vi "Open Talon Brtrfly v2.vi"() -> ()   [LabVIEW 2018]
uses:
  <vilib>/Rock Robotics/WPI/ThirdParty/Phoenix-LabVIEW/Motor Controller/Controls/CTRE_Phoenix_MotorControl_NeutralMode.ctl
  <vilib>/Rock Robotics/WPI/ThirdParty/Phoenix-LabVIEW/Motor Controller/Controls/CTRE_Phoenix_MotorControl_ControlMode.ctl
panel:
  out "Cursor.Cursor Position:Cursor Y":dbl
  out "Cursor.Cursor Position:Cursor X":dbl
  in  "Digital Joystick":cluster{"X":dbl, "Y":dbl}[](graph)
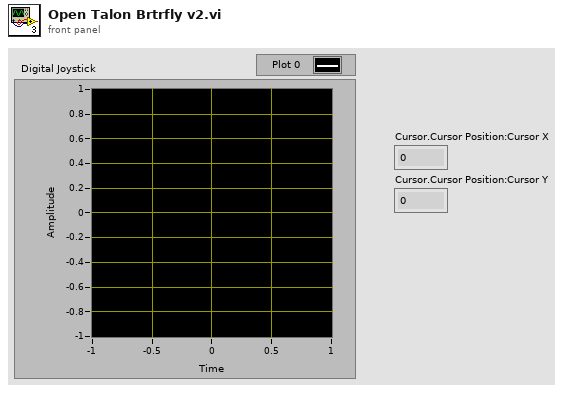
[diagram p1: front panel]
types:
  T1 = typedef "CTRE_Phoenix_MotorControl_ControlMode.ctl" = u16
  T2 = typedef "CTRE_Phoenix_MotorControl_NeutralMode.ctl" = enum8{"EEPROMSetting", "Override to Coast", "Override to Brake"}
  T3 = enum16{"FollowerType_PercentOutput", "FollowerType_AuxOutput1"}
  T4 = typedef "WPI_MotorControlDeviceRef.ctl" = cluster{"DeviceStatus":errorcluster, "Type":T5, "PWM":cluster{"PWM Channel":T6, "DeadBand":T7}, "CAN":cluster{"Device Number":u8, "SetOutput VI Ref":variant, "GetOutput VI Ref":variant, "Enable VI Ref":variant, "Disable VI Ref":variant, "Data":variant}, "Invert":bool, "DIO PWM":cluster{"PWM \"Enable\" Channel":T6, "DIOChannel":T8, "PWM Rate":dbl}}
  T5 = typedef "WPI_MotorControlType.ctl" = enum16{"PWM", "CAN", "DIO PWM"}
  T6 = typedef "FPGA_DIOPWMChannel.ctl" = enum8{"PWM 0", "PWM 1", "PWM 2", "PWM 3", "PWM 4", "PWM 5", "PWM 6", "PWM 7", "PWM 8", "PWM 9", "PWM MXP 0", "PWM MXP 1", "PWM MXP 2", "PWM MXP 3", "PWM MXP 4", "PWM MXP 5", "PWM MXP 6", "PWM MXP 7", "PWM MXP 8", "PWM MXP 9", "Invalid"}
  T7 = typedef "WPI_PWMDeadband.ctl" = cluster{"Name":string, "maxPositivePwm":i32, "minPositivePwm":i32, "centerPwm":i32, "maxNegativePwm":i32, "minNegativePwm":i32, "angularRange":u16}
  T8 = typedef "FPGA_DIOChannel.ctl" = enum8{"DIO 0", "DIO 1", "DIO 2", "DIO 3", "DIO 4", "DIO 5", "DIO 6", "DIO 7", "DIO 8", "DIO 9", "DIO MXP 0", "DIO MXP 1", "DIO MXP 2", "DIO MXP 3", "DIO MXP 4", "DIO MXP 5", "DIO MXP 6", "DIO MXP 7", "DIO MXP 8", "DIO MXP 9", "DIO MXP 10", "DIO MXP 11", "DIO MXP 12", "DIO MXP 13", "DIO MXP 14", "DIO MXP 15", "SPI Port CS1", "SPI Port CS2", "SPI Port CS3", "SPI Port MISO", "SPI Port MOSI", "Invalid"}
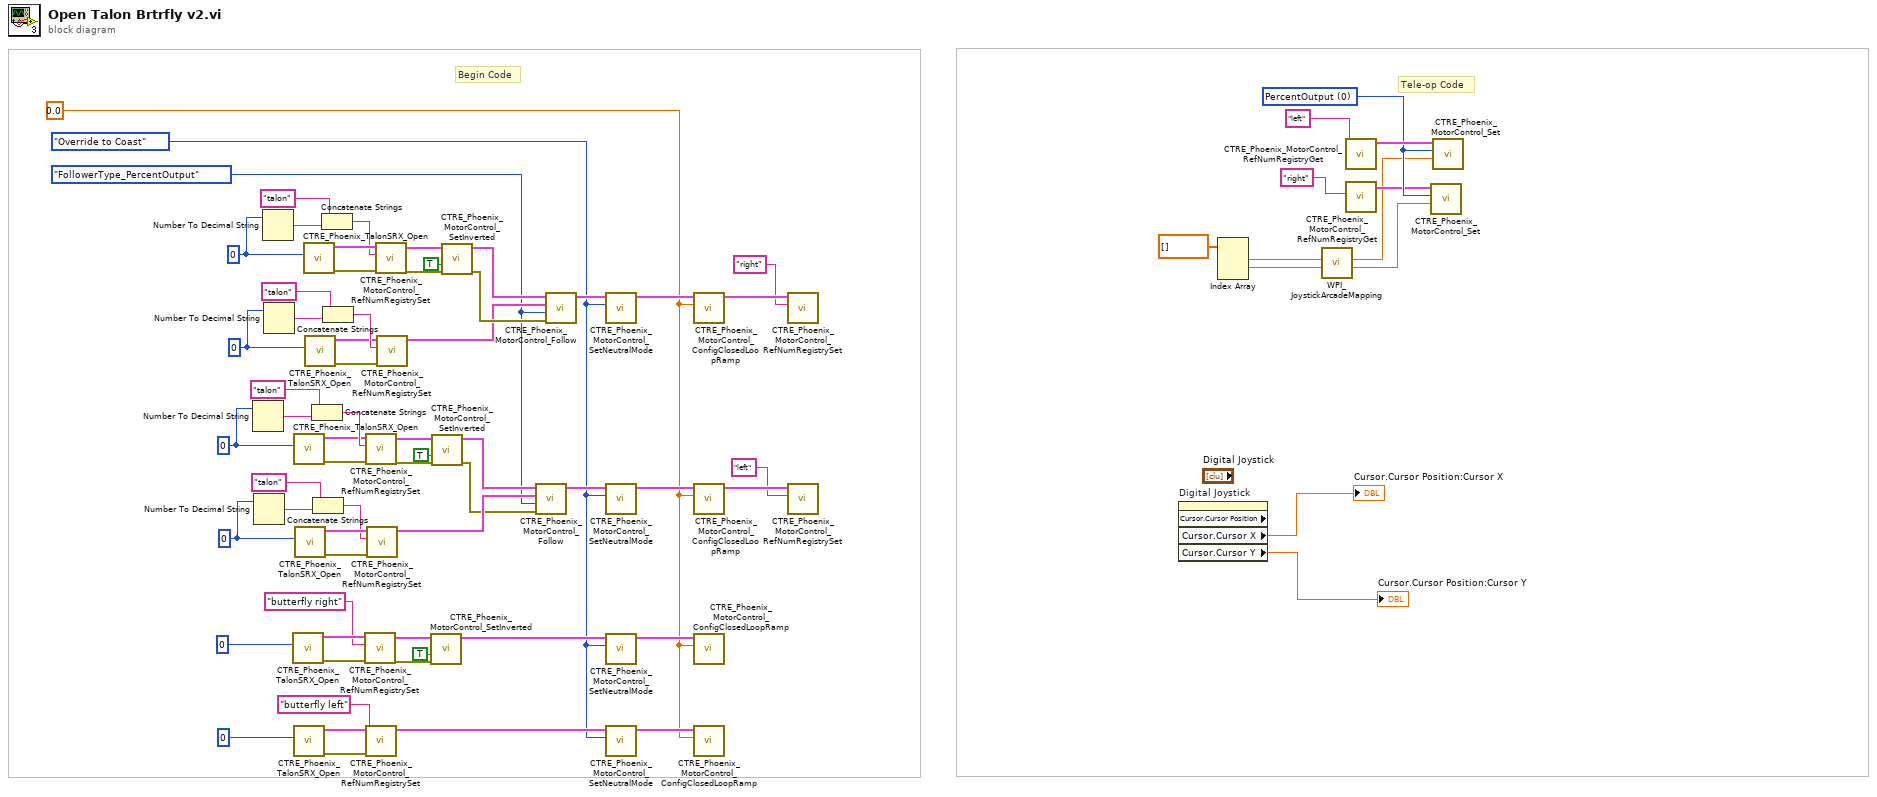
[diagram p0: block diagram]
diagram:
  w14 = T1 0 items=["PercentOutput"=0, "Position"=1, "Velocity"=2, "Current"=3, "Follower"=5, "MotionProfile"=6, "MotionMagic"=7, "MotionProfileArc"=10, "Disabled"=15] ("Control Mode")
  w2 = 0.0 ("secondsFromNeutralToFull")
  w1 = CTRE_Phoenix_MotorControl_NeutralMode."Override to Coast" ("Motor Control Neutral Mode")
  w25 = T3."FollowerType_PercentOutput" ("FollowerType")
  w47 = u8 0 ("Device Number")
  w40 = u8 0 ("Device Number")
  w62 = u8 0 ("Device Number")
  w69 = u8 0 ("Device Number")
  # "Tele-op Code"
  # "Begin Code"
  n1 = Number To Decimal String(number=w40) -> (decimal integer string=w41:string)  [unwired: 1 in]
  n2 = Number To Decimal String(number=w47) -> (decimal integer string=w46:string)  [unwired: 1 in]
  n3 = Number To Decimal String(number=w69) -> (decimal integer string=w68:string)  [unwired: 1 in]
  n4 = Number To Decimal String(number=w62) -> (decimal integer string=w63:string)  [unwired: 1 in]
  n5 = call <vilib>:"CTRE_Phoenix_TalonSRX_Open.vi"("Device Number"=u8 0) -> ("error out"=w33:errorcluster, "CAN Talon SRX Ref"=w32:T4)  [unwired: 9 in]
  n6 = call <vilib>:"CTRE_Phoenix_TalonSRX_Open.vi"("Device Number"=w40) -> ("error out"=w38:errorcluster, "CAN Talon SRX Ref"=w39:T4)  [unwired: 9 in]
  n7 = call <vilib>:"CTRE_Phoenix_TalonSRX_Open.vi"("Device Number"=u8 0) -> ("error out"=w28:errorcluster, "CAN Talon SRX Ref"=w29:T4)  [unwired: 9 in]
  n8 = call <vilib>:"CTRE_Phoenix_TalonSRX_Open.vi"("Device Number"=w47) -> ("error out"=w49:errorcluster, "CAN Talon SRX Ref"=w48:T4)  [unwired: 9 in]
  n9 = call <vilib>:"CTRE_Phoenix_TalonSRX_Open.vi"("Device Number"=w69) -> ("error out"=w71:errorcluster, "CAN Talon SRX Ref"=w70:T4)  [unwired: 9 in]
  n10 = call <vilib>:"CTRE_Phoenix_TalonSRX_Open.vi"("Device Number"=w62) -> ("error out"=w60:errorcluster, "CAN Talon SRX Ref"=w61:T4)  [unwired: 9 in]
  n11 = Concatenate Strings("talon" ("string"), w41) -> (w43:string)
  n12 = Concatenate Strings("talon" ("string"), w46) -> (w44:string)
  n13 = Concatenate Strings("talon" ("string"), w68) -> (w66:string)
  n14 = Concatenate Strings("talon" ("string"), w63) -> (w65:string)
  n15 = call <vilib>:"CTRE_Phoenix_MotorControl_RefNumRegistrySet.vi"("error in (no error)"=w33, "refnum name"="butterfly right", "PhoenixMotorControlDevRef"=w32) -> ("error out"=w26:errorcluster, "PhoenixMotorControlDevRef"=w27:T4)  [unwired: 7 in]
  n16 = call <vilib>:"CTRE_Phoenix_MotorControl_RefNumRegistrySet.vi"("error in (no error)"=w38, "refnum name"=w43, "PhoenixMotorControlDevRef"=w39) -> ("error out"=w51:errorcluster, "PhoenixMotorControlDevRef"=w50:T4)  [unwired: 7 in]
  n17 = call <vilib>:"CTRE_Phoenix_MotorControl_RefNumRegistrySet.vi"("error in (no error)"=w28, "refnum name"="butterfly left", "PhoenixMotorControlDevRef"=w29) -> ("PhoenixMotorControlDevRef"=w5:T4)  [unwired: 7 in, 1 out]
  n18 = call <vilib>:"CTRE_Phoenix_MotorControl_RefNumRegistrySet.vi"("error in (no error)"=w49, "refnum name"=w44, "PhoenixMotorControlDevRef"=w48) -> ("PhoenixMotorControlDevRef"=w54:T4)  [unwired: 7 in, 1 out]
  n19 = call <vilib>:"CTRE_Phoenix_MotorControl_RefNumRegistrySet.vi"("error in (no error)"=w71, "refnum name"=w66, "PhoenixMotorControlDevRef"=w70) -> ("error out"=w58:errorcluster, "PhoenixMotorControlDevRef"=w59:T4)  [unwired: 7 in]
  n20 = call <vilib>:"CTRE_Phoenix_MotorControl_RefNumRegistrySet.vi"("error in (no error)"=w60, "refnum name"=w65, "PhoenixMotorControlDevRef"=w61) -> ("PhoenixMotorControlDevRef"=w55:T4)  [unwired: 7 in, 1 out]
  n21 = call <vilib>:"CTRE_Phoenix_MotorControl_SetInverted.vi"("error in (no error)"=w26, "Invert?"=TRUE, "PhoenixMotorControlDevRef"=w27) -> ("PhoenixMotorControlDevRef"=w6:T4)  [unwired: 7 in, 1 out]
  n22 = call <vilib>:"CTRE_Phoenix_MotorControl_SetInverted.vi"("error in (no error)"=w51, "Invert?"=TRUE, "PhoenixMotorControlDevRef"=w50) -> ("error out"=w52:errorcluster, "PhoenixMotorControlDevRef"=w53:T4)  [unwired: 7 in]
  n23 = call <vilib>:"CTRE_Phoenix_MotorControl_SetInverted.vi"("error in (no error)"=w58, "Invert?"=TRUE, "PhoenixMotorControlDevRef"=w59) -> ("error out"=w57:errorcluster, "PhoenixMotorControlDevRef"=w56:T4)  [unwired: 7 in]
  n24 = call <vilib>:"CTRE_Phoenix_MotorControl_Follow.vi"("error in (no error)"=w52, "FollowerType"=w25, "Master Controller to Follow"=w54, "PhoenixMotorControlDevRef"=w53) -> ("PhoenixMotorControlDevRef"=w36:T4)  [unwired: 6 in, 1 out]
  n25 = call <vilib>:"CTRE_Phoenix_MotorControl_Follow.vi"("error in (no error)"=w57, "FollowerType"=w25, "Master Controller to Follow"=w55, "PhoenixMotorControlDevRef"=w56) -> ("PhoenixMotorControlDevRef"=w73:T4)  [unwired: 6 in, 1 out]
  n26 = call <vilib>:"CTRE_Phoenix_MotorControl_SetNeutralMode.vi"("Motor Control Neutral Mode"=w1, "PhoenixMotorControlDevRef"=w73) -> ("PhoenixMotorControlDevRef"=w72:T4)  [unwired: 8 in, 1 out]
  n27 = call <vilib>:"CTRE_Phoenix_MotorControl_SetNeutralMode.vi"("Motor Control Neutral Mode"=w1, "PhoenixMotorControlDevRef"=w36) -> ("PhoenixMotorControlDevRef"=w37:T4)  [unwired: 8 in, 1 out]
  n28 = call <vilib>:"CTRE_Phoenix_MotorControl_SetNeutralMode.vi"("Motor Control Neutral Mode"=w1, "PhoenixMotorControlDevRef"=w6) -> ("PhoenixMotorControlDevRef"=w3:T4)  [unwired: 8 in, 1 out]
  n29 = call <vilib>:"CTRE_Phoenix_MotorControl_SetNeutralMode.vi"("Motor Control Neutral Mode"=w1, "PhoenixMotorControlDevRef"=w5) -> ("PhoenixMotorControlDevRef"=w4:T4)  [unwired: 8 in, 1 out]
  n30 = call <vilib>:"CTRE_Phoenix_MotorControl_ConfigClosedLoopRamp.vi"("secondsFromNeutralToFull"=w2, "PhoenixMotorControlDevRef"=w72) -> ("PhoenixMotorControlDevRef"=w24:T4)  [unwired: 8 in, 1 out]
  n31 = call <vilib>:"CTRE_Phoenix_MotorControl_ConfigClosedLoopRamp.vi"("secondsFromNeutralToFull"=w2, "PhoenixMotorControlDevRef"=w37) -> ("PhoenixMotorControlDevRef"=w23:T4)  [unwired: 8 in, 1 out]
  n32 = call <vilib>:"CTRE_Phoenix_MotorControl_ConfigClosedLoopRamp.vi"("secondsFromNeutralToFull"=w2, "PhoenixMotorControlDevRef"=w3) -> ()  [unwired: 8 in, 2 out]
  n33 = call <vilib>:"CTRE_Phoenix_MotorControl_ConfigClosedLoopRamp.vi"("secondsFromNeutralToFull"=w2, "PhoenixMotorControlDevRef"=w4) -> ()  [unwired: 8 in, 2 out]
  n34 = call <vilib>:"CTRE_Phoenix_MotorControl_RefNumRegistrySet.vi"("refnum name"="right", "PhoenixMotorControlDevRef"=w24) -> ()  [unwired: 8 in, 2 out]
  n35 = call <vilib>:"CTRE_Phoenix_MotorControl_RefNumRegistrySet.vi"("refnum name"="left", "PhoenixMotorControlDevRef"=w23) -> ()  [unwired: 8 in, 2 out]
  n36 = property on="Digital Joystick" class="XYGraph (strict)" props=["Cursor", "Cursor Position", "Cursor", "Cursor X", "Cursor", "Cursor Y"]() -> ("Cursor.Cursor X"=→"Cursor.Cursor Position:Cursor X":dbl, "Cursor.Cursor Y"=→"Cursor.Cursor Position:Cursor Y":dbl)  [unwired: 2 in, 3 out]
  n37 = Index Array(array=dbl[] []) -> (element #1=w19:dbl, element #2=w18:dbl)  [unwired: 3 in, 1 out]
  n38 = call <vilib>:"WPI_JoystickArcadeMapping.vi"("Y axis value"=w18, "X axis value"=w19) -> ("Right Motor Value"=w11:dbl, "Left Motor Value"=w12:dbl)  [unwired: 8 in]
  n39 = call <vilib>:"CTRE_Phoenix_MotorControl_RefNumRegistryGet.vi"("refnum name"="left") -> ("PhoenixMotorControlDevRef"=w15:T4)  [unwired: 9 in, 1 out]
  n40 = call <vilib>:"CTRE_Phoenix_MotorControl_RefNumRegistryGet.vi"("refnum name"="right") -> ("PhoenixMotorControlDevRef"=w13:T4)  [unwired: 9 in, 1 out]
  n41 = call <vilib>:"CTRE_Phoenix_MotorControl_Set.vi"("Output"=w11, "Control Mode"=w14, "PhoenixMotorControlDevRef"=w13) -> ()  [unwired: 7 in, 2 out]
  n42 = call <vilib>:"CTRE_Phoenix_MotorControl_Set.vi"("Output"=w12, "Control Mode"=w14, "PhoenixMotorControlDevRef"=w15) -> ()  [unwired: 7 in, 2 out]
